vi "c_Insert About View.vi"() -> (1 "Case Label":T1)   [LabVIEW 2018, in "Main View.lvclass"]
uses:
  Main View.lvclass
  <vilib>/addons/_Workers/Library/Case Label.ctl
  <vilib>/addons/_Workers/Library/Workers.lvlib
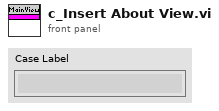
[diagram p1: front panel]
types:
  T1 = typedef "Workers.lvlib/Case Label.ctl" = string
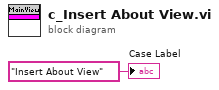
[diagram p0: block diagram]
diagram:
  "Case Label" <- T1 "Insert About View" ("Case Label")
